vi "PlanckExperiment_Main.vi"() -> ()   [LabVIEW 2015]
uses:
  <vilib>/Instr/_visa.llb/VISA Configure Serial Port (Instr).vi
panel:
  out "灯丝的本次电流值(A) 2":dbl
  out "步进电机循环次数":dbl
  out "信号曲线":cluster{dbl[], "AD7606数组":dbl[]}[](graph)
  out "AD7606数组":dbl[](array[numeric])
  out "灯丝的本次电流值(A)":dbl
  in  "设定灯丝两端电压(V)":dbl[](array[numeric])
  out "AD7606当前电压值":dbl
  out "记录数据":bool=TRUE
  out "一次步进脉冲数":dbl
  in  "步进电机移动总长度(mm)":dbl=25.0
  in  "步进一次的距离(mm)":dbl=0.25
  out "电源串口状态灯":bool
  in  "flow control (0:none) 2":u16(ring) caption="流控制（0:无）" items=["无", "XON/XOFF", "RTS/CTS", "XON/XOFF & RTS/CTS", "DTR/DSR", "XON/XOFF & DTR/DSR"]
  in  "stop bits (10: 1 bit) 2":u16=10 caption="停止位（10: 1位）"
  in  "波特率(默认9600)":u32=9600
  in  "奇偶 (0:none) 2":enum16{"None", "Odd", "Even", "Mark", "Space"}(ring) caption="奇偶（0:无）"
  in  "数据比特(默认8)":u16(ring)=8 items=["5"=5, "6"=6, "7"=7, "8"=8]
  in  "电源端口":refnum<visa-resource-name>="COM1"
  out "记录的接收":string
  out "ARM板串口状态灯":bool
  out "接收":string
  in  "flow control (0:none)":u16(ring) caption="流控制（0:无）" items=["无", "XON/XOFF", "RTS/CTS", "XON/XOFF & RTS/CTS", "DTR/DSR", "XON/XOFF & DTR/DSR"]
  in  "stop bits (10: 1 bit)":u16=10 caption="停止位（10: 1位）"
  in  "波特率(默认9600)":u32=9600
  in  "停止":bool
  in  "开始":bool
  in  "奇偶 (0:none)":enum16{"None", "Odd", "Even", "Mark", "Space"}(ring) caption="奇偶（0:无）"
  in  "数据比特(默认8)":u16(ring)=8 items=["5"=5, "6"=6, "7"=7, "8"=8]
  in  "ARM板端口":refnum<visa-resource-name>="COM1"
  # "串口调试助手状态机\n三部分组成：\n1、状态机本身（枚举）\n①界面初始化\n②打开串口\n③等待用户触发（读取、写入）\n④关闭串口\n⑤退出\n2、选择分支\n3、While循环结构（重点移位寄存器）"
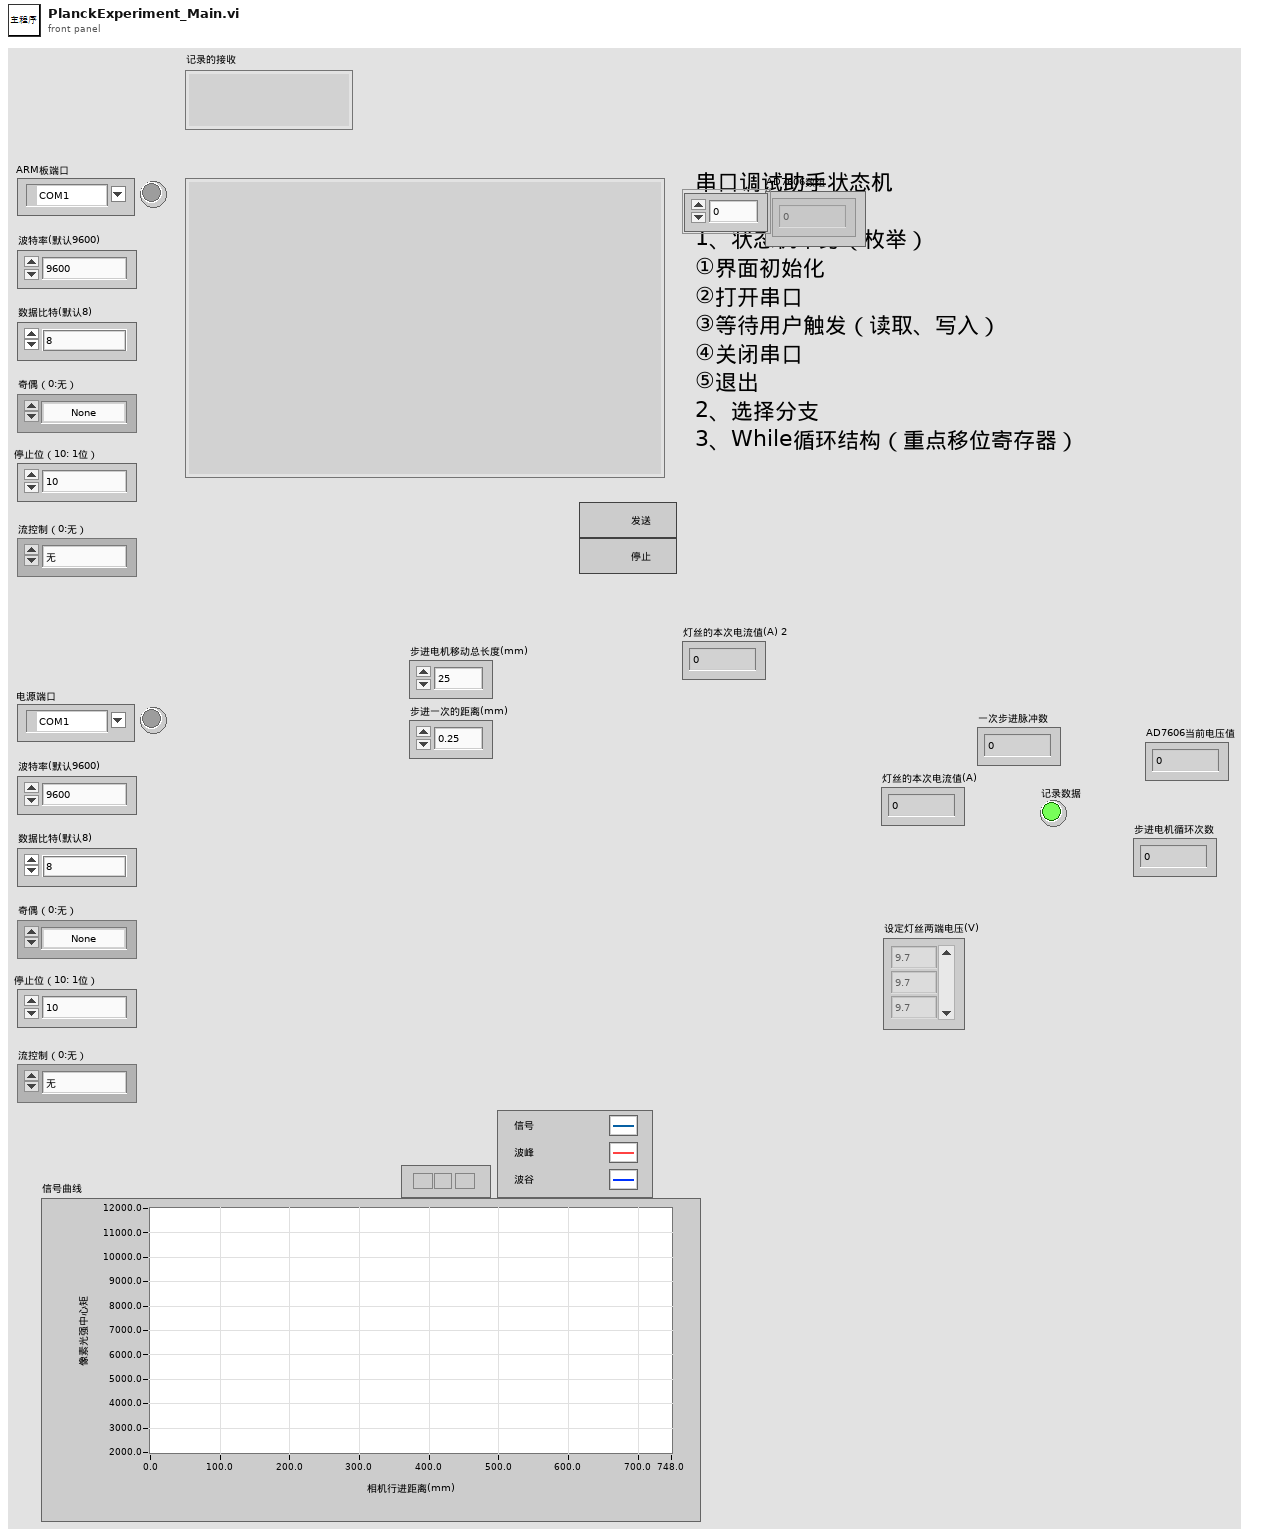
[diagram p1: front panel]
types:
  T1 = typedef "状态机.ctl" = enum16{"初始化_包含电机参数初始化", "打开串口", "电源设定", "电源参数读取", "等待用户触发", "读取", "曲线图像处理和寻峰", "写入_发送步进指令", "步进电机回退", "关闭串口", "退出"}
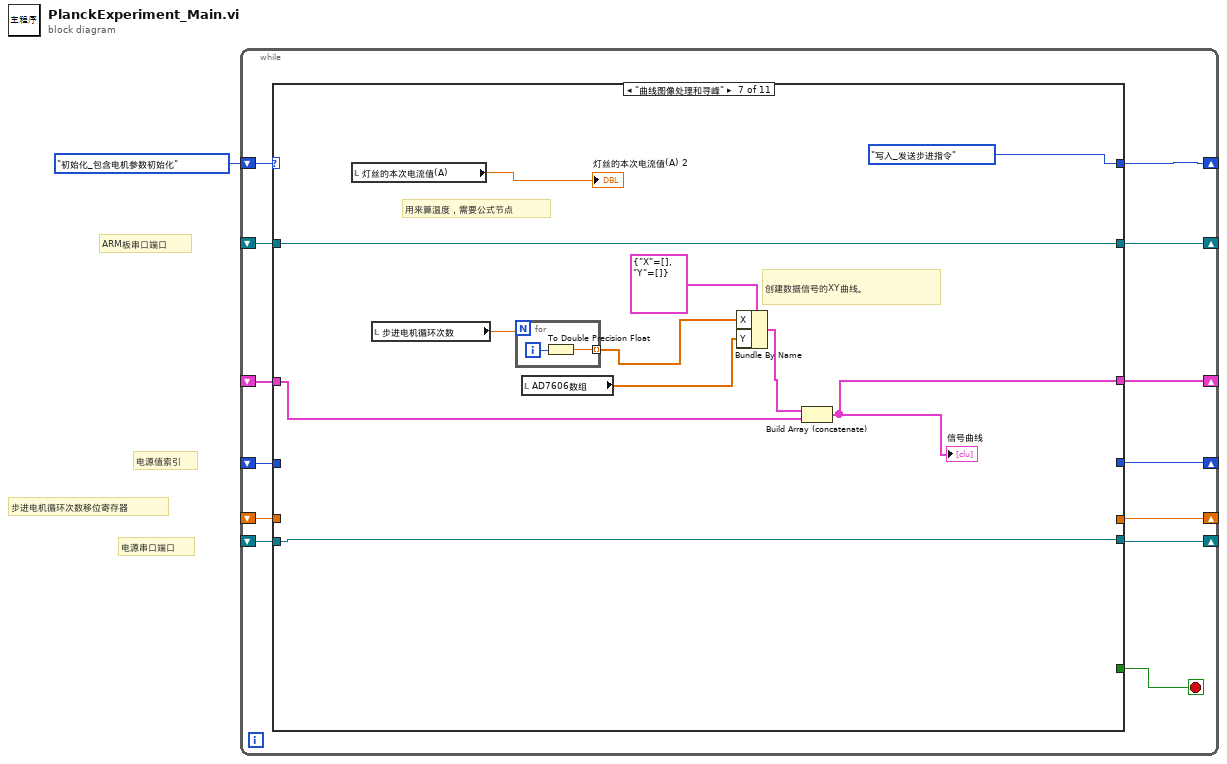
[diagram p0: block diagram]
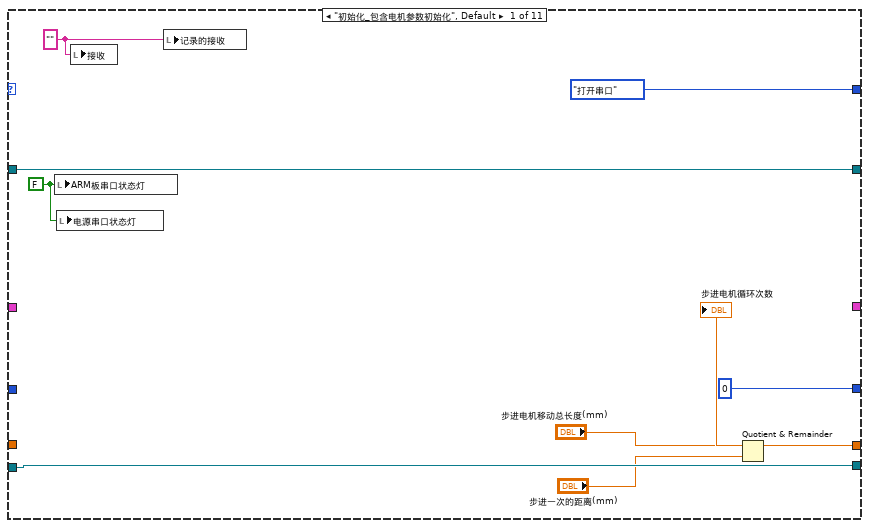
[diagram p2: hidden frame]
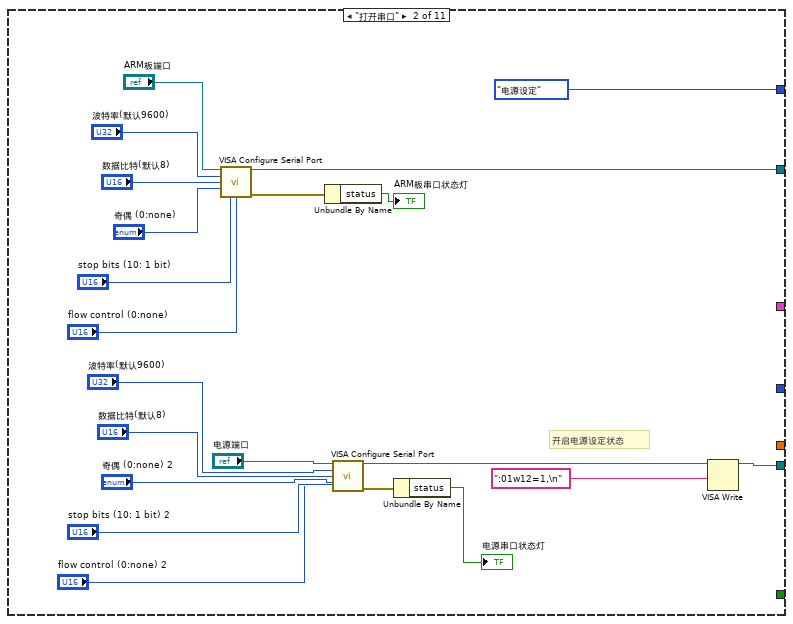
[diagram p3: hidden frame]
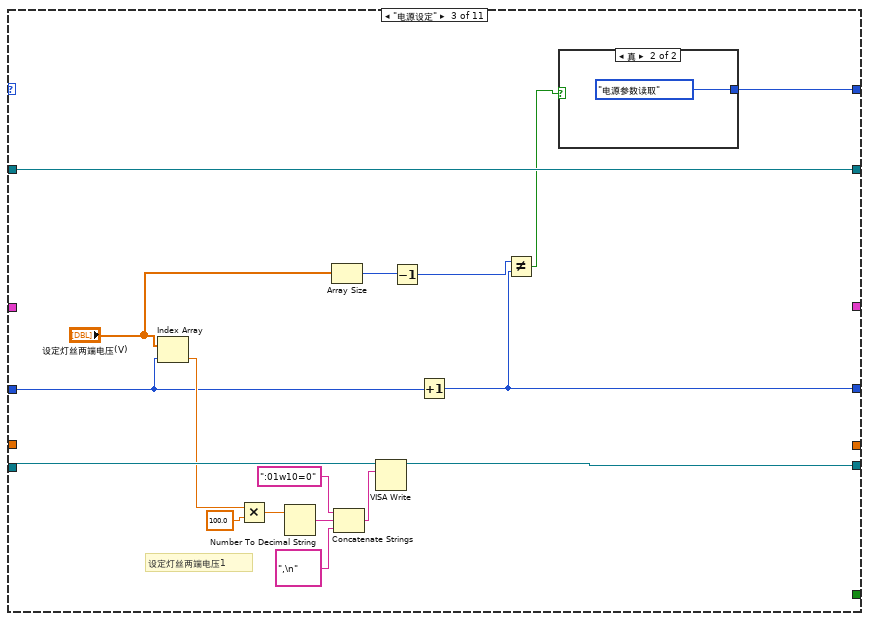
[diagram p4: hidden frame]
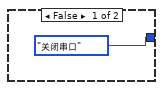
[diagram p5: hidden frame]
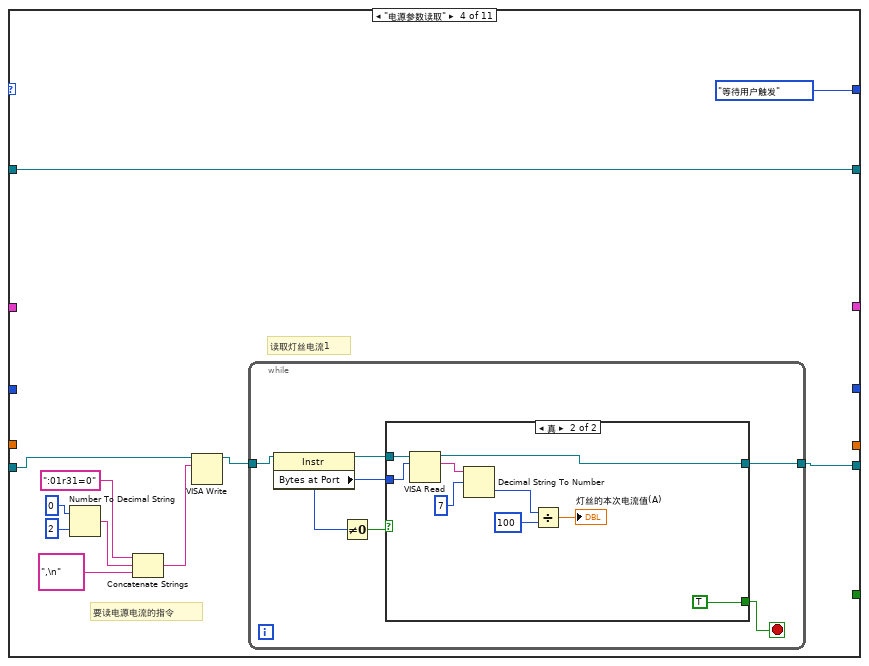
[diagram p6: hidden frame]
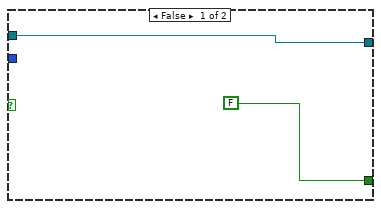
[diagram p7: hidden frame]
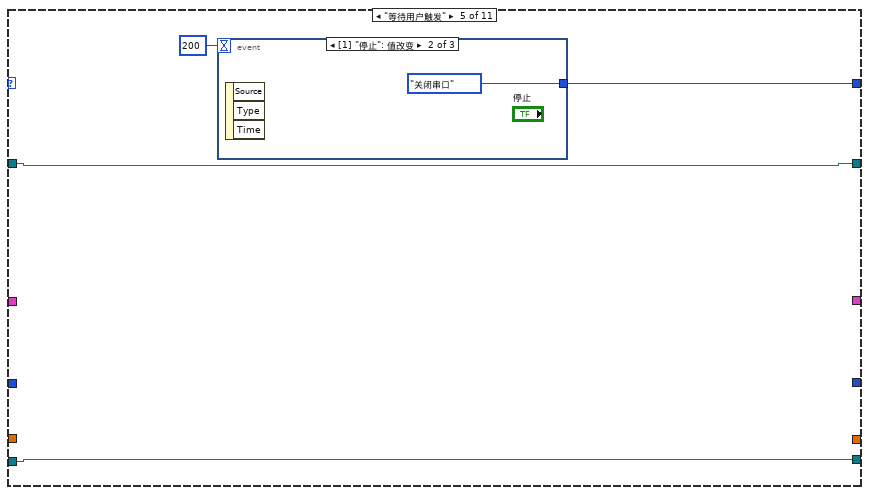
[diagram p8: hidden frame]
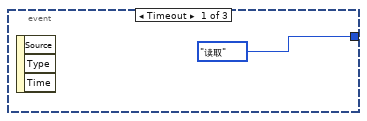
[diagram p9: hidden frame]
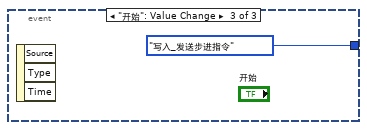
[diagram p10: hidden frame]
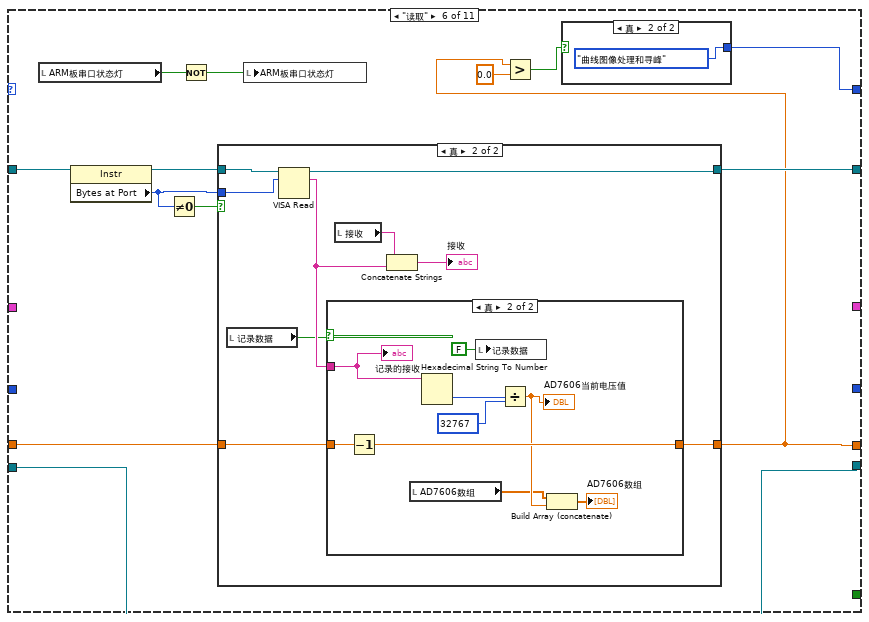
[diagram p11: hidden frame]
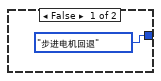
[diagram p12: hidden frame]
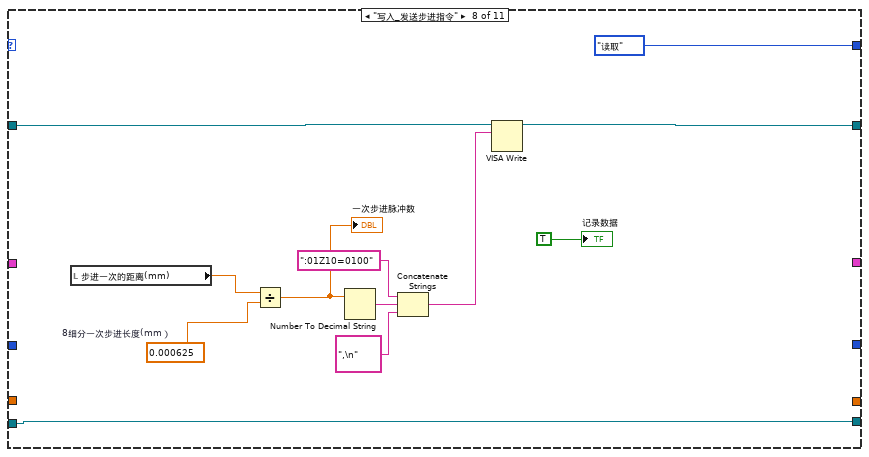
[diagram p15: hidden frame]
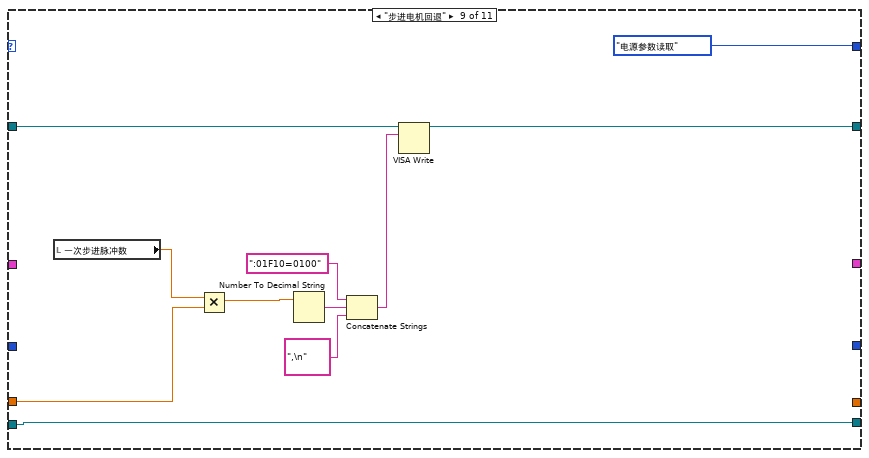
[diagram p16: hidden frame]
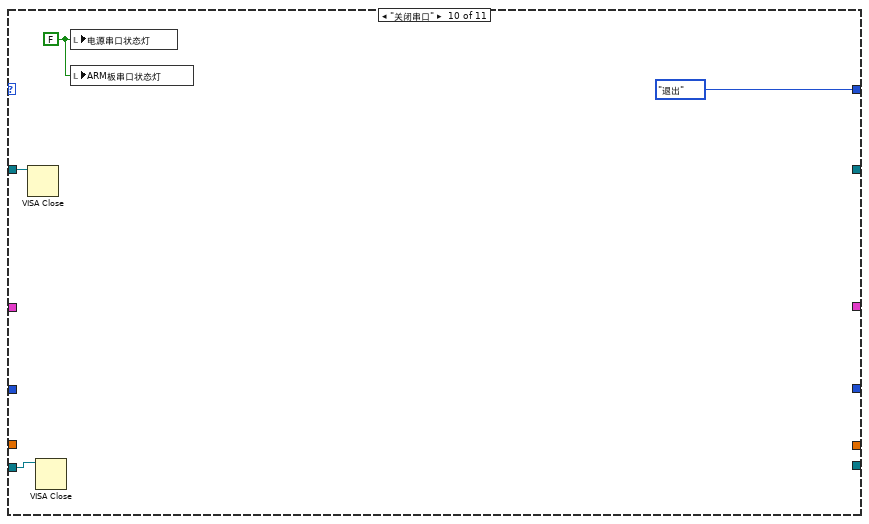
[diagram p17: hidden frame]
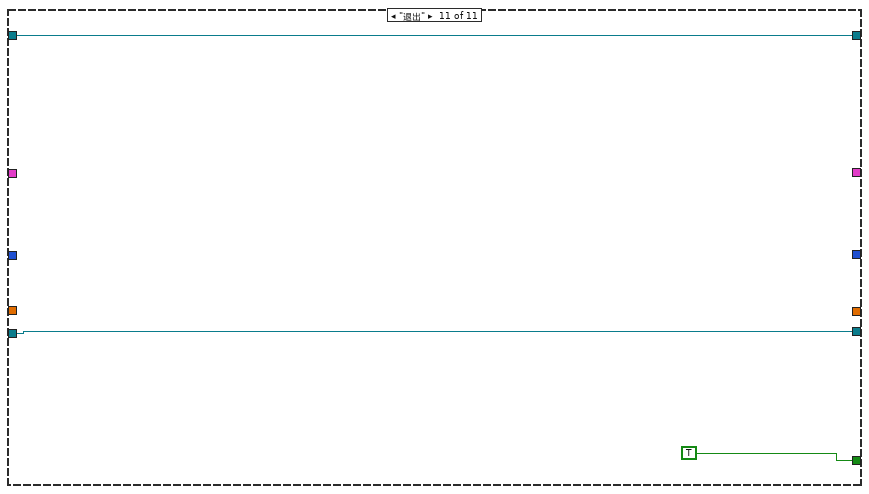
[diagram p18: hidden frame]
diagram:
  # "电源串口端口"
  # "ARM板串口端口"
  # "步进电机循环次数移位寄存器"
  # "电源值索引"
  n1 = while {
    shift-right: [w13] -> _
    shift-left: 状态机."初始化_包含电机参数初始化" ("状态机") -> [w14]
    shift-right: [w11] -> _
    shift-left: _ -> [w10]
    shift-right: [w9] -> _
    shift-left: _ -> [w8]
    shift-right: [w7] -> _
    shift-left: _ -> [w6]
    shift-right: [w4] -> _
    shift-left: _ -> [w5]
    shift-right: [w2] -> _
    shift-left: _ -> [w3]
    stop <- w12 stop-if-true
    n2 = case shown="\"曲线图像处理和寻峰\"" w14 {
      tunnel: [状态机."打开串口" ("状态机") 状态机."电源设定" ("状态机") w60 状态机."等待用户触发" ("状态机") w95 w111 状态机."写入_发送步进指令" ("状态机") 状态机."读取" ("状态机") 状态机."电源参数读取" ("状态机") 状态机."退出" ("状态机") _] -> w13
      tunnel: [_ _ _ _ _ _ _ _ _ _ TRUE] -> w12
      tunnel: [w22 w37 w61 w74 w93 w110 w143 w148 w159 _ w174] -> w11
      tunnel: w10 -> [w22 _ w61 w74 w93 w109 w143 w146 w160 w171 w174]
      tunnel: [w20 w24 w58 w67 w92 w103 w142 w156 w168 _ w173] -> w9
      tunnel: w8 -> [w20 _ w59 w68 w92 w103 w142 w156 w168 w169 w173]
      tunnel: [w18 _ _ _ _ w100 _ _ _ _ _] -> w7
      tunnel: w6 -> [_ _ _ _ _ w102 _ _ w166 _ _]
      tunnel: w5 -> [_ _ w50 _ _ _ _ _ _ _ _]
      tunnel: [0 ("索引") _ w46 _ _ _ _ _ _ _ _] -> w4
      tunnel: w3 -> [_ _ _ _ _ _ w137 _ _ _ _]
      tunnel: [_ _ _ _ _ _ w138 _ _ _ _] -> w2
      frame "初始化_包含电机参数初始化", Default {
        w21 = "" ("接收")
        w19 = FALSE ("串口状态灯")
        n3 = local write "ARM板串口状态灯"(w19) -> ()
        n4 = local write "电源串口状态灯"(w19) -> ()
        n5 = local write "接收"(w21) -> ()
        n6 = local write "记录的接收"(w21) -> ()
        n7 = Quotient & Remainder(x="步进电机移动总长度(mm)", y="步进一次的距离(mm)") -> (x-y*floor(x/y)=w18:dbl)  [unwired: 1 out]
        "步进电机循环次数" <- w18
      }
      frame "打开串口" {
        # "开启电源设定状态"
        n8 = call-poly "VISA Configure Serial Port"("VISA resource name"="ARM板端口", "baud rate (9600)"="波特率(默认9600)", "data bits (8)"="数据比特(默认8)", "parity (0:none)"="奇偶 (0:none)", "stop bits (10: 1 bit)"="stop bits (10: 1 bit)", "flow control (0:none)"="flow control (0:none)") -> ("VISA resource name out"=w37:refnum<visa-resource-name>, "error out"=w36:errorcluster)  [unwired: 8 in]
        n9 = Unbundle By Name(w36) -> ("status"=→"ARM板串口状态灯":bool)
        n10 = call-poly "VISA Configure Serial Port"("VISA resource name"="电源端口", "baud rate (9600)"="波特率(默认9600)", "data bits (8)"="数据比特(默认8)", "parity (0:none)"="奇偶 (0:none) 2", "stop bits (10: 1 bit)"="stop bits (10: 1 bit) 2", "flow control (0:none)"="flow control (0:none) 2") -> ("VISA resource name out"=w25:refnum<visa-resource-name>, "error out"=w28:errorcluster)  [unwired: 8 in]
        n11 = Unbundle By Name(w28) -> ("status"=→"电源串口状态灯":bool)
        n12 = VISA Write(VISA resource name=w25, write buffer=":01w12=1,\n") -> (VISA resource name out=w24:refnum<visa-resource-name>)  [unwired: 1 in, 2 out]
      }
      frame "电源设定" {
        # "设定灯丝两端电压1"
        n13 = Index Array(array="设定灯丝两端电压(V)", index=w50) -> (element=w51:dbl)
        n14 = Multiply(x=w51, y=100.0) -> (x*y=w57:dbl)
        n15 = Number To Decimal String(number=w57) -> (decimal integer string=w55:string)  [unwired: 1 in]
        n16 = Array Size(array="设定灯丝两端电压(V)") -> (size(s)=w48:i32)
        n17 = Concatenate Strings(":01w10=0", w55, ",\n") -> (w52:string)
        n18 = VISA Write(VISA resource name=w59, write buffer=w52) -> (VISA resource name out=w58:refnum<visa-resource-name>)  [unwired: 1 in, 2 out]
        n19 = Decrement(x=w48) -> (x-1=w47:i32)
        n20 = Increment(x=w50) -> (x+1=w46:i32)
        n21 = Not Equal?(x=w47, y=w46) -> (x != y?=w45:bool)
        n22 = case shown="真" w45 {
          tunnel: [状态机."关闭串口" ("状态机") 状态机."电源参数读取" ("状态机")] -> w60
          frame False {
          }
          frame True {
          }
        }
      }
      frame "电源参数读取" {
        # "要读电源电流的指令"
        # "读取灯丝电流1"
        n23 = Number To Decimal String(number=0, width (-)=i16 2 ("宽度(-)")) -> (decimal integer string=w73:string)
        n24 = Concatenate Strings(":01r31=0", w73, ",\n") -> (w69:string)
        n25 = VISA Write(VISA resource name=w68, write buffer=w69) -> (VISA resource name out=w66:refnum<visa-resource-name>)  [unwired: 1 in, 2 out]
        n26 = while {
          tunnel: w66 -> [w79]
          tunnel: [w80] -> w67
          stop <- w76 stop-if-true
          n27 = property class="Instr"(reference=w79) -> (reference out=w78:refnum<visa-resource-name>, "Bytes at Port"=w75:u32)  [unwired: 1 in, 1 out]
          n28 = Not Equal To 0?(x=w75) -> (x != 0?=w77:bool)
          n29 = case shown="真" w77 {
            tunnel: [w82 w87] -> w80
            tunnel: w78 -> [w82 w86]
            tunnel: [FALSE TRUE] -> w76
            tunnel: w75 -> [_ w84]
            frame False {
            }
            frame True {
              n30 = VISA Read(VISA resource name=w86, byte count=w84) -> (VISA resource name out=w87:refnum<visa-resource-name>, read buffer=w89:string)  [unwired: 1 in, 2 out]
              n31 = Decimal String To Number(string=w89, offset=7 ("偏移量")) -> (number=w90:i32)  [unwired: 1 in, 1 out]
              n32 = Divide(x=w90, y=100) -> (x/y=→"灯丝的本次电流值(A)":dbl)
            }
          }
        }
      }
      frame "等待用户触发" {
        n33 = event shown="[1] \"停止\": 值改变" {
          selector: _ -> [_ _ _]
          dyn-events: _ -> [_ _ _]
          timeout: 200 -> [_ _ _]
          tunnel: [状态机."读取" ("状态机") 状态机."关闭串口" ("状态机") 状态机."写入_发送步进指令" ("状态机")] -> w95
          event Timeout {
            n34 = event-data() -> ()  [unwired: 1 in, 3 out]
          }
          event "停止": Value Change {
            n35 = event-data() -> ()  [unwired: 1 in, 3 out]
          }
          event "开始": Value Change {
            n36 = event-data() -> ()  [unwired: 1 in, 3 out]
          }
        }
      }
      frame "读取" {
        n37 = local read "ARM板串口状态灯"() -> (w105:bool)
        n38 = property class="Instr"(reference=w109) -> (reference out=w108:refnum<visa-resource-name>, "Bytes at Port"=w106:u32)  [unwired: 1 in, 1 out]
        n39 = Not Equal To 0?(x=w106) -> (x != 0?=w107:bool)
        n40 = Not(x=w105) -> (.not. x?=w104:bool)
        n41 = case shown="真" w107 {
          tunnel: [w114 w123] -> w110
          tunnel: w108 -> [w114 w122]
          tunnel: w106 -> [_ w121]
          tunnel: w102 -> [_ w116]
          tunnel: [_ w115] -> w100
          frame False {
          }
          frame True {
            n42 = local read "记录数据"() -> (w117:bool)
            n43 = VISA Read(VISA resource name=w122, byte count=w121) -> (VISA resource name out=w123:refnum<visa-resource-name>, read buffer=w118:string)  [unwired: 1 in, 2 out]
            n44 = case shown="真" w117 {
              tunnel: w118 -> [_ w131]
              tunnel: w116 -> [_ w128]
              tunnel: [_ w127] -> w115
              frame False {
              }
              frame True {
                n45 = Decrement(x=w128) -> (x-1=w127:dbl)
                n46 = local read "AD7606数组"() -> (w124:dbl[])
                n47 = Hexadecimal String To Number(string=w131) -> (number=w130:u32)  [unwired: 2 in, 1 out]
                n48 = local write "记录数据"(FALSE ("记录数据")) -> ()
                n49 = Divide(x=w130, y=u32 32767) -> (x/y=w126:dbl)
                "AD7606当前电压值" <- w126
                n50 = Build Array (concatenate)(w124, w126) -> (→"AD7606数组":dbl[])
                "记录的接收" <- w131
              }
            }
            n51 = local read "接收"() -> (w120:string)
            n52 = Concatenate Strings(w120, w118) -> (→"接收":string)
          }
        }
        n53 = local write "ARM板串口状态灯"(w104) -> ()
        n54 = Greater?(x=w100, y=0.0) -> (0:w99:bool)
        n55 = case shown="真" w99 {
          tunnel: [状态机."步进电机回退" ("状态机") 状态机."曲线图像处理和寻峰" ("状态机")] -> w111
          frame False {
          }
          frame True {
          }
        }
      }
      frame "曲线图像处理和寻峰" {
        # "用来算温度，需要公式节点"
        # "创建数据信号的XY曲线。"
        n56 = local read "灯丝的本次电流值(A)"() -> (→"灯丝的本次电流值(A) 2":dbl)
        n57 = local read "步进电机循环次数"() -> (w140:dbl)
        n58 = for {
          N: w140 -> [_]
          tunnel: [w144] -> w136 mode=indexing
          i -> [w145]
          n59 = To Double Precision Float(number=w145) -> (double precision float=w144:dbl)
        }
        n60 = local read "AD7606数组"() -> (w135:dbl[])
        n61 = Bundle By Name(cluster=cluster{"X":dbl[], "Y":dbl[]} {"X"=[], "Y"=[]} ("输入簇"), "X"=w136, "Y"=w135) -> (w133:cluster{"X":dbl[], "Y":dbl[]})
        n62 = Build Array (concatenate)(w133, w137) -> (w138:cluster{"X":dbl[], "Y":dbl[]}[])
        "信号曲线" <- w138
      }
      frame "写入_发送步进指令" {
        w149 = 0.000625  # 8细分一次步进长度(mm）
        n63 = local read "步进一次的距离(mm)"() -> (w150:dbl)
        n64 = Divide(x=w150, y=w149) -> (x/y=w154:dbl)
        "一次步进脉冲数" <- w154
        n65 = Number To Decimal String(number=w154) -> (decimal integer string=w155:string)  [unwired: 1 in]
        n66 = Concatenate Strings(":01Z10=0100", w155, ",\n") -> (w152:string)
        n67 = VISA Write(VISA resource name=w146, write buffer=w152) -> (VISA resource name out=w148:refnum<visa-resource-name>)  [unwired: 1 in, 2 out]
        "记录数据" <- TRUE
      }
      frame "步进电机回退" {
        n68 = local read "一次步进脉冲数"() -> (w167:dbl)
        n69 = Multiply(x=w167, y=w166) -> (x*y=w161:dbl)
        n70 = Number To Decimal String(number=w161) -> (decimal integer string=w162:string)  [unwired: 1 in]
        n71 = Concatenate Strings(":01F10=0100", w162, ",\n") -> (w164:string)
        n72 = VISA Write(VISA resource name=w160, write buffer=w164) -> (VISA resource name out=w159:refnum<visa-resource-name>)  [unwired: 1 in, 2 out]
      }
      frame "关闭串口" {
        w170 = FALSE ("串口状态灯")
        n73 = VISA Close(VISA resource name=w171) -> ()  [unwired: 1 in, 1 out]
        n74 = VISA Close(VISA resource name=w169) -> ()  [unwired: 1 in, 1 out]
        n75 = local write "电源串口状态灯"(w170) -> ()
        n76 = local write "ARM板串口状态灯"(w170) -> ()
      }
      frame "退出" {
      }
    }
  }
